vi "Audio_Transformation_Setted_Frequency_v009.vi"() -> ()   [LabVIEW 2019]
uses:
  <vilib>/sound2/lvsound2.llb/Sound Data Format.ctl
  <vilib>/sound2/lvsound2.llb/Sound Input Read (DBL).vi
  <vilib>/addons/Time Frequency Analysis/Transform.llb/TFA Online Gabor Transform (Real).vi
  <vilib>/addons/_Advanced Signal Processing/NI_AdvSigProcTFA.lvlib
panel:
  out "u(t)":T1(graph)
  out "V(t)":T1(graph)
  out "Noise Speech":dbl[](graph)
  in  "Address selector":i32[](array[numeric])
  in  "Neuron Type":T2(ring)
  out "max index(es)":i32
  out "max value":dbl
  out "Waveform Graph":dbl[](graph)
  out "Magnitude of Gabor Coefficients":dbl[][](graph)
  in  "Stop":bool
  # "Step two : Graph of the amplitude of the Gabor coefficient of the different bins"
  # "Step three : Spike Response of the neurons"
  # "Step one: Sound recorded from the computer"
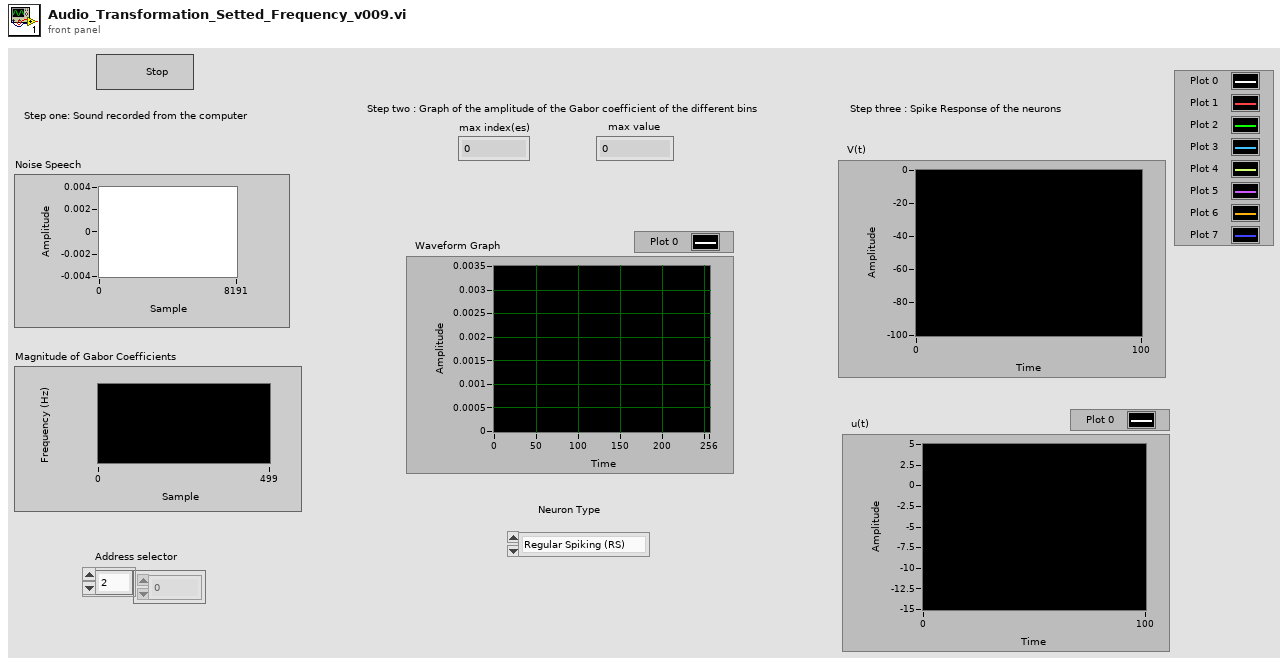
[diagram p1: front panel]
types:
  T1 = cluster{"[0]":dbl, "[1]":dbl, "[2]":dbl, "[3]":dbl, "[4]":dbl, "[5]":dbl, "[6]":dbl, "[7]":dbl}
  T2 = enum16{"Regular Spiking (RS)", "Intrinsically Bursting (IB)", "Chattering (CH)", "Fast Spiking (FS)", "Thalamo-Cortical 1 (TC1)", "Thalamo-Cortical 2 (TC2)", "Resonator (RZ)", "Low-Threshold Spiking (LTS)", "Phasic Spiking (PS)"}
  T3 = typedef "Sound Data Format.ctl" = cluster{"sample rate (S/s)":dbl, "number of channels":i32, "bits per sample":i32}
  T4 = cluster{"analysis window":dbl[], "dM (time steps)":i32, "N (frequency bins)":i32}
  T5 = typedef "Sound Input Task ID.ctl" = u32
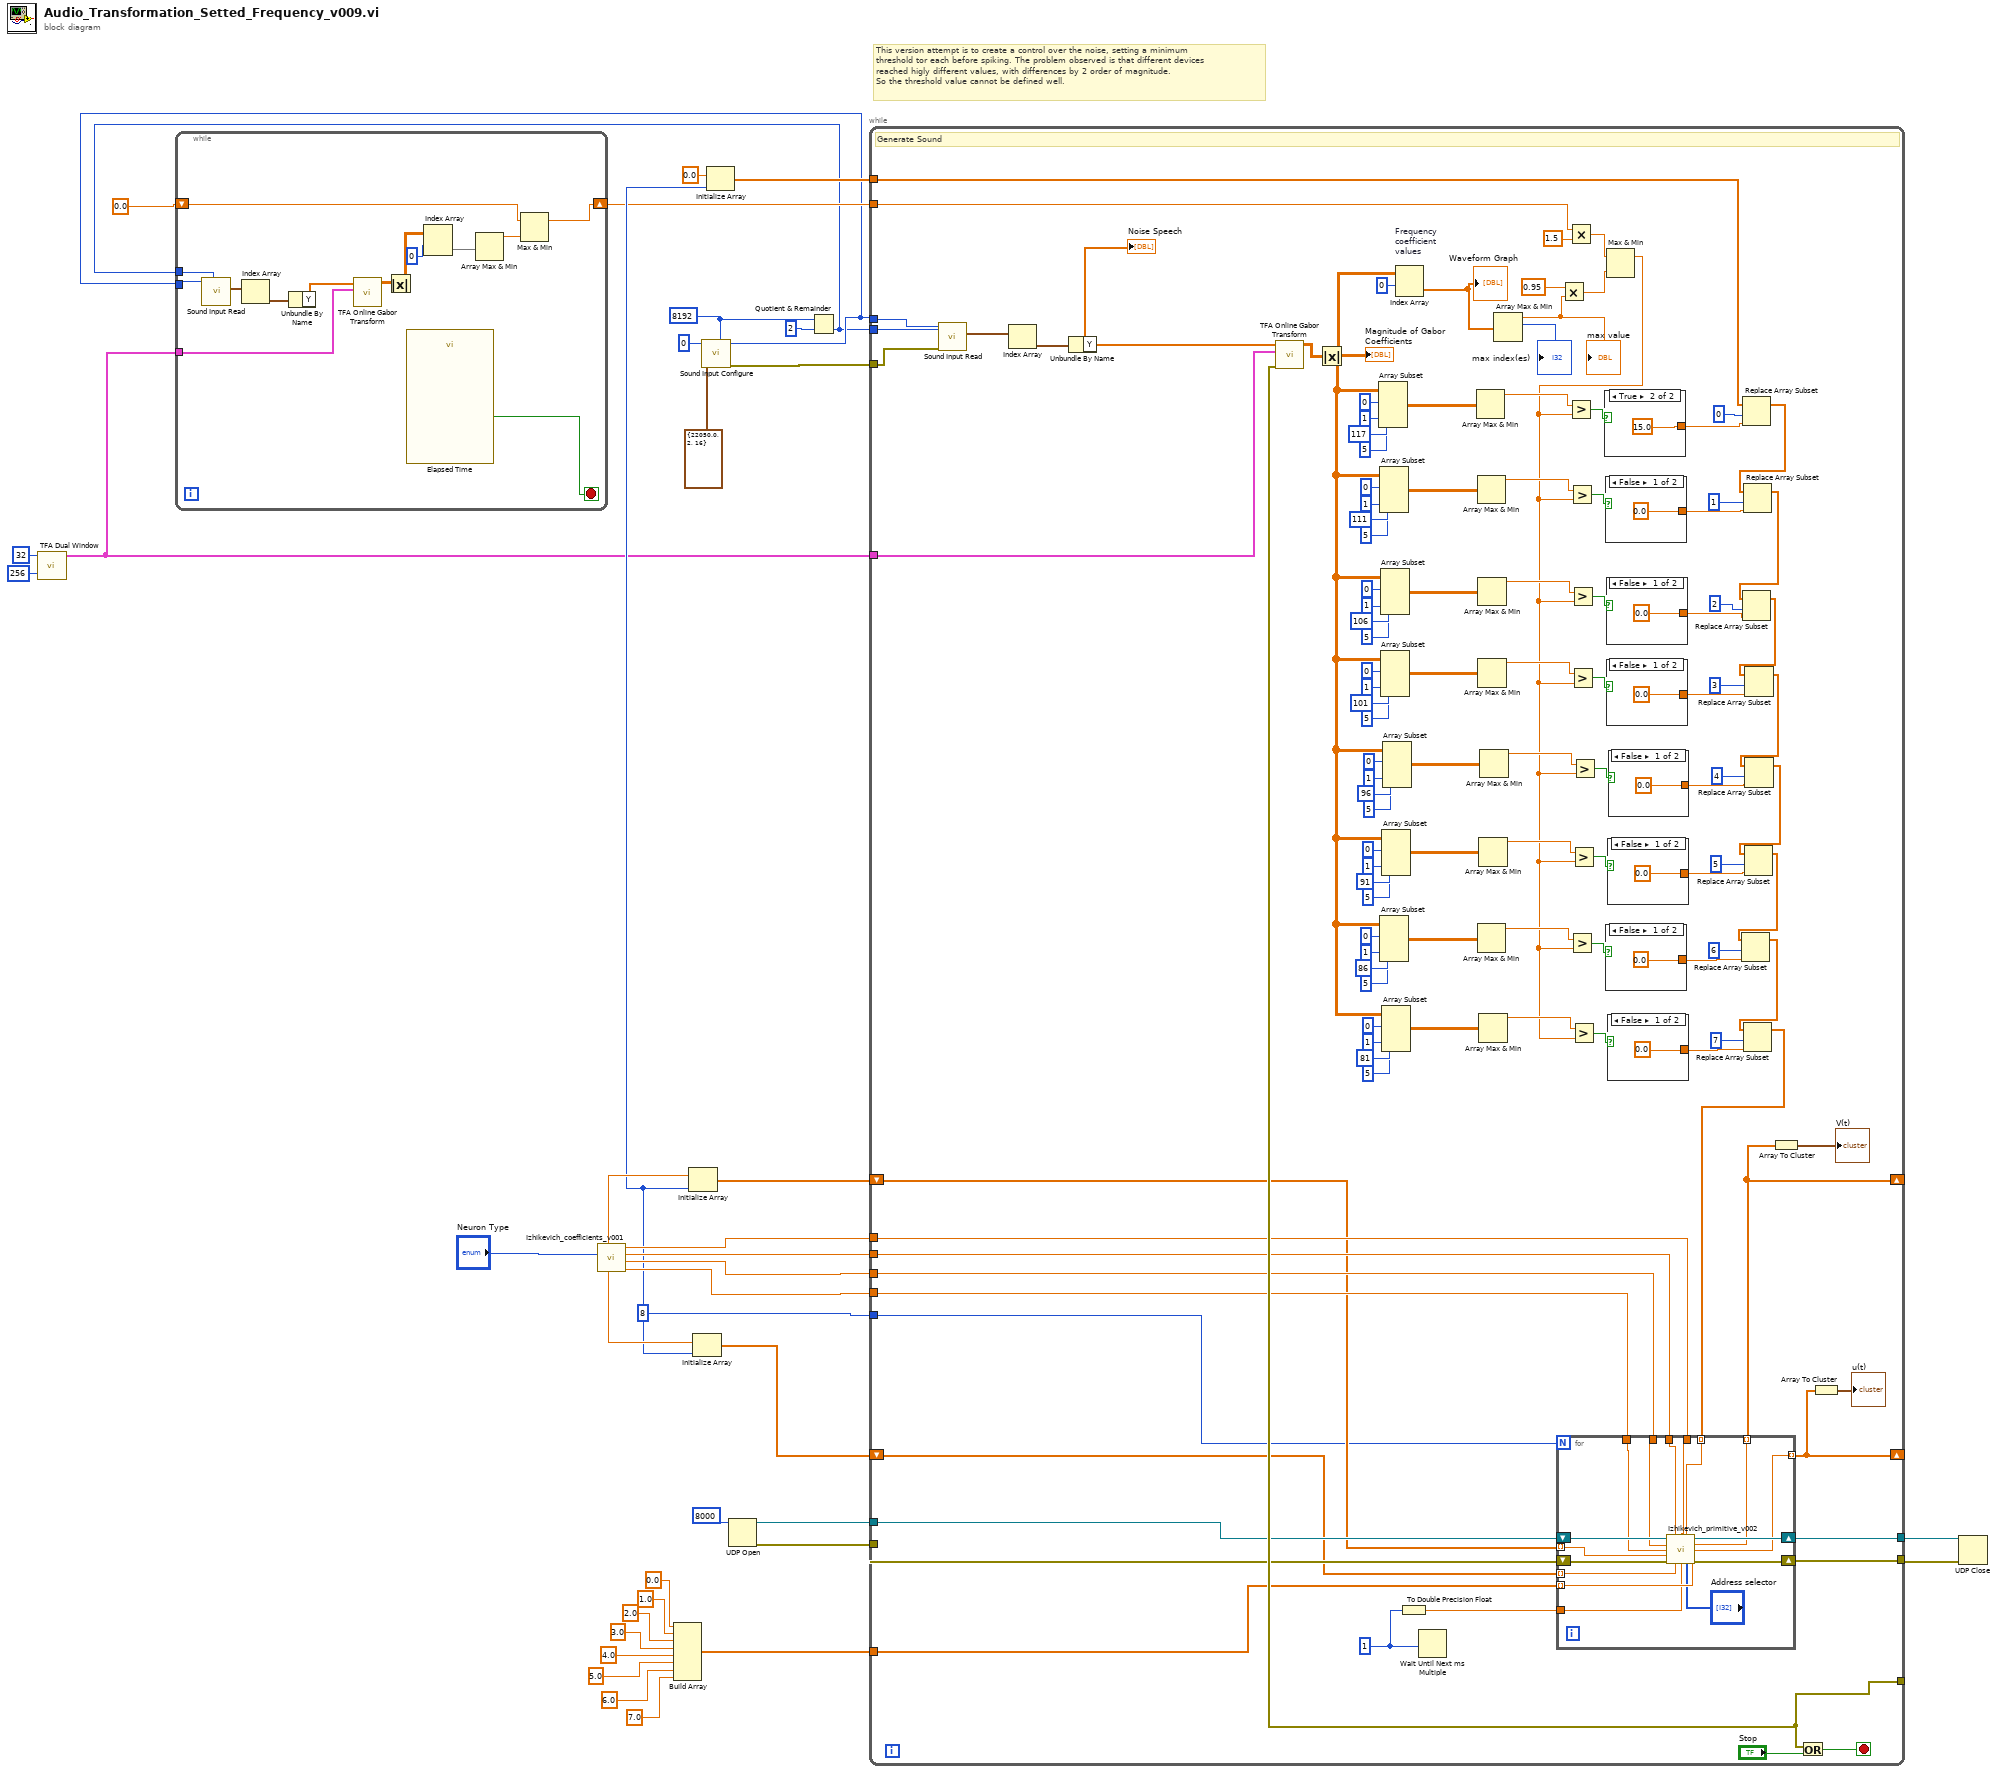
[diagram p0: block diagram]
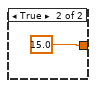
[diagram p2: hidden frame]
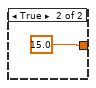
[diagram p3: hidden frame]
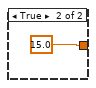
[diagram p4: hidden frame]
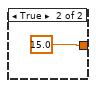
[diagram p5: hidden frame]
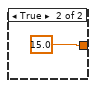
[diagram p6: hidden frame]
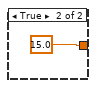
[diagram p7: hidden frame]
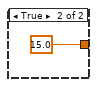
[diagram p8: hidden frame]
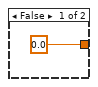
[diagram p9: hidden frame]
diagram:
  w17 = 8
  w24 = 8192 ("number of samples/ch")
  # "This version attempt is to create a control over the noise, setting a minimum\nthreshold tor each before spiking. The problem observed is that different devices\nreached higly different values, with differences by 2 order of magnitude.\nSo the threshold value cannot be defined well."
  n1 = call <vilib>:"TFA Dual Window.vi"("N (frequency bins)"=256, "dM (time steps)"=32) -> ("analysis info"=w14:T4)  [unwired: 7 in, 2 out]
  n2 = call "Izhikevich_coefficients_v001.vi"("Neuron Type"="Neuron Type") -> ("d"=w32:dbl, "c"=w33:dbl, "b"=w34:dbl, "a"=w35:dbl, "u0"=w19:dbl, "v0"=w21:dbl)  [unwired: 3 in]
  n3 = Build Array(0.0 ("element"), 1.0 ("element"), 2.0 ("element"), 3.0 ("element"), 4.0 ("element"), 5.0 ("element"), 6.0 ("element"), 7.0 ("element")) -> (w1:dbl[])
  n4 = Initialize Array(w21, w17) -> (w20:dbl[])
  n5 = Initialize Array(w19, w17) -> (w18:dbl[])
  n6 = call <vilib>:"Sound Input Configure.vi"("number of samples/ch"=w24, "sound format"=T3 {"sample rate (S/s)"=22050.0, "number of channels"=2, "bits per sample"=16}, "device ID"=u32 0) -> ("error out"=w22:errorcluster, "task ID"=w11:T5)  [unwired: 7 in]
  n7 = Initialize Array(0.0 ("element"), w17) -> (w15:dbl[])
  n8 = UDP Open(11:u16 8000 ("port")) -> (port=w30:refnum<k16>, 0:w29:errorcluster)  [unwired: 4 in, 1 out]
  n9 = Quotient & Remainder(x=w24, y=2) -> (floor(x/y)=w10:i32)  [unwired: 1 out]
  n10 = while {
    tunnel: w14 -> [w50]
    shift-right: [w42] -> w12
    shift-left: 0.0 -> [w43]
    tunnel: w11 -> [w40]
    tunnel: w10 -> [w39]
    stop <- w41 stop-if-true
    n11 = call-poly <vilib>:"Sound Input Read.vi"("number of samples/ch"=w39, "task ID"=w40) -> ("data"=w51:waveform(dbl)[])  [unwired: 7 in, 2 out]
    n12 = Index Array(array=w51) -> (element=w52:waveform(dbl))  [unwired: 1 in]
    n13 = Unbundle By Name(w52) -> ("Y"=w49:dbl[])
    n14 = call-poly <vilib>:"TFA Online Gabor Transform.vi"("transform info"=w50, "signal"=w49) -> ("Gabor coef"=w48:cdb[][])  [unwired: 7 in, 2 out]
    n15 = Absolute Value(x=w48) -> (abs(x)=w46:dbl[][])
    n16 = call "Elapsed Time"() -> ("Time has Elapsed"=w41:bool)  [unwired: 12 in, 7 out]
    n17 = Index Array(array=w46, index (row)=0) -> (element=w45:dbl[])  [unwired: 1 in]
    n18 = Array Max & Min(array=w45) -> (max value=w44:dbl)  [unwired: 3 out]
    n19 = Max & Min(x=w43, y=w44) -> (max(x,y)=w42:dbl)  [unwired: 1 out]
  }
  n20 = while {
    tunnel: [w166] -> _
    tunnel: w14 -> [w171]
    shift-right: [w54] -> _
    shift-left: w20 -> [w155]
    shift-right: [w53] -> _
    shift-left: w18 -> [w154]
    tunnel: w35 -> [w165]
    tunnel: w34 -> [w164]
    tunnel: w33 -> [w162]
    tunnel: w32 -> [w161]
    tunnel: w30 -> [w163]
    tunnel: w29 -> [w160]
    tunnel: [w157] -> w28
    tunnel: [w156] -> w27
    tunnel: w11 -> [w152]
    tunnel: w22 -> [w151]
    tunnel: w10 -> [w153]
    tunnel: w17 -> [w147]
    tunnel: w15 -> [w119]
    tunnel: w12 -> [w60]
    tunnel: w1 -> [w55]
    stop <- w172 stop-if-true
    w159 = u32 1 ("millisecond multiple")
    # "Generate Sound"
    n21 = call-poly <vilib>:"Sound Input Read.vi"("number of samples/ch"=w153, "error in (no error)"=w151, "task ID"=w152) -> ("data"=w149:waveform(dbl)[])  [unwired: 6 in, 2 out]
    n22 = Index Array(array=w149) -> (element=w150:waveform(dbl))  [unwired: 1 in]
    n23 = Unbundle By Name(w150) -> ("Y"=w148:dbl[])
    "Noise Speech" <- w148
    n24 = call-poly <vilib>:"TFA Online Gabor Transform.vi"("transform info"=w171, "signal"=w148) -> ("error out"=w166:errorcluster, "Gabor coef"=w170:cdb[][])  [unwired: 7 in, 1 out]
    n25 = Absolute Value(x=w170) -> (abs(x)=w67:dbl[][])
    "Magnitude of Gabor Coefficients" <- w67
    n26 = Array Subset(array=w67, index (row)=0 ("index"), length (row)=1 ("length"), index (col)=117 ("index"), length (col)=5 ("length")) -> (w142:dbl[][])
    n27 = Array Subset(array=w67, index (row)=0 ("index"), length (row)=1 ("length"), index (col)=111 ("index"), length (col)=5 ("length")) -> (w135:dbl[][])
    n28 = Array Subset(array=w67, index (row)=0 ("index"), length (row)=1 ("length"), index (col)=86 ("index"), length (col)=5 ("length")) -> (w82:dbl[][])
    n29 = Array Subset(array=w67, index (row)=0 ("index"), length (row)=1 ("length"), index (col)=106 ("index"), length (col)=5 ("length")) -> (w124:dbl[][])
    n30 = Array Subset(array=w67, index (row)=0 ("index"), length (row)=1 ("length"), index (col)=101 ("index"), length (col)=5 ("length")) -> (w112:dbl[][])
    n31 = Array Subset(array=w67, index (row)=0 ("index"), length (row)=1 ("length"), index (col)=91 ("index"), length (col)=5 ("length")) -> (w92:dbl[][])
    n32 = Array Subset(array=w67, index (row)=0 ("index"), length (row)=1 ("length"), index (col)=81 ("index"), length (col)=5 ("length")) -> (w72:dbl[][])
    n33 = Array Subset(array=w67, index (row)=0 ("index"), length (row)=1 ("length"), index (col)=96 ("index"), length (col)=5 ("length")) -> (w102:dbl[][])
    n34 = Index Array "Frequency \ncoefficient \nvalues"(array=w67, index (row)=0) -> (element=w168:dbl[])  [unwired: 1 in]
    "Waveform Graph" <- w168
    n35 = To Double Precision Float(number=w159) -> (double precision float=w158:dbl)
    n36 = Wait Until Next ms Multiple(millisecond multiple=w159) -> ()  [unwired: 1 out]
    n37 = Array Max & Min(array=w142) -> (max value=w141:dbl)  [unwired: 3 out]
    n38 = Array Max & Min(array=w135) -> (max value=w134:dbl)  [unwired: 3 out]
    n39 = Array Max & Min(array=w82) -> (max value=w81:dbl)  [unwired: 3 out]
    n40 = Array Max & Min(array=w124) -> (max value=w123:dbl)  [unwired: 3 out]
    n41 = Array Max & Min(array=w112) -> (max value=w111:dbl)  [unwired: 3 out]
    n42 = Array Max & Min(array=w92) -> (max value=w91:dbl)  [unwired: 3 out]
    n43 = Array Max & Min(array=w72) -> (max value=w71:dbl)  [unwired: 3 out]
    n44 = Array Max & Min(array=w102) -> (max value=w101:dbl)  [unwired: 3 out]
    n45 = Array Max & Min(array=w168) -> (max value=w57:dbl, max index (indices)=→"max index(es)":i32)  [unwired: 2 out]
    "max value" <- w57
    n46 = Multiply(x=0.95 ("y"), y=w57) -> (x*y=w58:dbl)
    n47 = Multiply(x=w60, y=1.5) -> (x*y=w59:dbl)
    n48 = Max & Min(x=w59, y=w58) -> (max(x,y)=w62:dbl)  [unwired: 1 out]
    n49 = Greater?(x=w141, y=w62) -> (0:w140:bool)
    n50 = Greater?(x=w134, y=w62) -> (0:w133:bool)
    n51 = Greater?(x=w81, y=w62) -> (0:w80:bool)
    n52 = Greater?(x=w123, y=w62) -> (0:w122:bool)
    n53 = Greater?(x=w111, y=w62) -> (0:w110:bool)
    n54 = Greater?(x=w91, y=w62) -> (0:w90:bool)
    n55 = Greater?(x=w71, y=w62) -> (0:w70:bool)
    n56 = Greater?(x=w101, y=w62) -> (0:w100:bool)
    n57 = case shown="True" w140 {
      tunnel: [0.0 15.0] -> w132
      frame False {
      }
      frame True {
      }
    }
    n58 = case shown="False" w133 {
      tunnel: [0.0 15.0] -> w129
      frame False {
      }
      frame True {
      }
    }
    n59 = case shown="False" w80 {
      tunnel: [0.0 15.0] -> w78
      frame False {
      }
      frame True {
      }
    }
    n60 = case shown="False" w122 {
      tunnel: [0.0 15.0] -> w120
      frame False {
      }
      frame True {
      }
    }
    n61 = case shown="False" w110 {
      tunnel: [0.0 15.0] -> w108
      frame False {
      }
      frame True {
      }
    }
    n62 = case shown="False" w90 {
      tunnel: [0.0 15.0] -> w88
      frame False {
      }
      frame True {
      }
    }
    n63 = case shown="False" w70 {
      tunnel: [0.0 15.0] -> w68
      frame False {
      }
      frame True {
      }
    }
    n64 = case shown="False" w100 {
      tunnel: [0.0 15.0] -> w98
      frame False {
      }
      frame True {
      }
    }
    n65 = Replace Array Subset(array=w119, new element=w132, index=0) -> (w118:dbl[])
    n66 = Replace Array Subset(array=w118, new element=w129, index=1) -> (w117:dbl[])
    n67 = Replace Array Subset(array=w117, new element=w120, index=2) -> (w107:dbl[])
    n68 = Replace Array Subset(array=w107, new element=w108, index=3) -> (w97:dbl[])
    n69 = Replace Array Subset(array=w97, new element=w98, index=4) -> (w87:dbl[])
    n70 = Replace Array Subset(array=w87, new element=w88, index=5) -> (w77:dbl[])
    n71 = Replace Array Subset(array=w77, new element=w78, index=6) -> (w66:dbl[])
    n72 = Replace Array Subset(array=w66, new element=w68, index=7) -> (w65:dbl[])
    n73 = for {
      N: w147 -> [_]
      tunnel: w165 -> [w194]
      tunnel: w164 -> [w195]
      tunnel: w162 -> [w196]
      tunnel: w161 -> [w197]
      tunnel: w158 -> [w200]
      tunnel: w155 -> [w203] mode=indexing
      tunnel: w154 -> [w202] mode=indexing
      shift-right: [w193] -> w156
      shift-left: w163 -> [w205]
      shift-right: [w192] -> w157
      shift-left: w160 -> [w204]
      tunnel: w65 -> [w198] mode=indexing
      tunnel: w55 -> [w201] mode=indexing
      tunnel: [w191] -> w54 mode=indexing
      tunnel: [w190] -> w53 mode=indexing
      n74 = call "Izhikevich_primitive_v002.vi"("UDP Network Connection in"=w205, "b"=w195, "a"=w194, "I"=w198, "c"=w196, "d"=w197, "v(t)"=w203, "error in (no error)"=w204, "u(t)"=w202, "Numeric"=w200, "Address selector"="Address selector", "Neuron ID"=w201) -> ("UDP Network Connection out"=w193:refnum<k16>, "v(t+dt)"=w191:dbl, "u(t+dt)"=w190:dbl, "error out"=w192:errorcluster)
    }
    n75 = Array To Cluster(array=w54) -> (cluster=→"V(t)":T1)
    n76 = Or(x=w166, y="Stop") -> (x .or. y?=w172:bool)
    n77 = Array To Cluster(array=w53) -> (cluster=→"u(t)":T1)
  }
  n78 = UDP Close(connection ID=w27, 8:w28) -> ()  [unwired: 2 out]
